vi "HEWH_Agilent_34972A.vi"(8 "error in":errorcluster, 11 "Message Queues out":T2) -> (0 "error out":errorcluster)   [LabVIEW 2023]
uses:
  Tenney/support/Message Queue/All Message Queues.ctl
  Tenney/support/Message Queue/Message Cluster.ctl
  Type Definitions/HEWH Agilent Data.ctl
  Type Definitions/HEWH Full Station IDs.ctl
  FVIR and LDO/support/Message Queue/Enqueue Message (Single).vi
  FVIR and LDO/support/Message Queue/Message Queue.lvlib
  Drivers/Agilent 34972/Agilent 34970.lvlib
  <vilib>/Utility/error.llb/whitespace.ctl
  Tenney/support/Message Queue/Tenney Message Queue.lvlib
panel:
  out "Debug":string[](array[string])
  in  "Debug":bool
  out "Agilent Data":T1
  out "Analog Channel-List":string
  out "Loop Count":i32
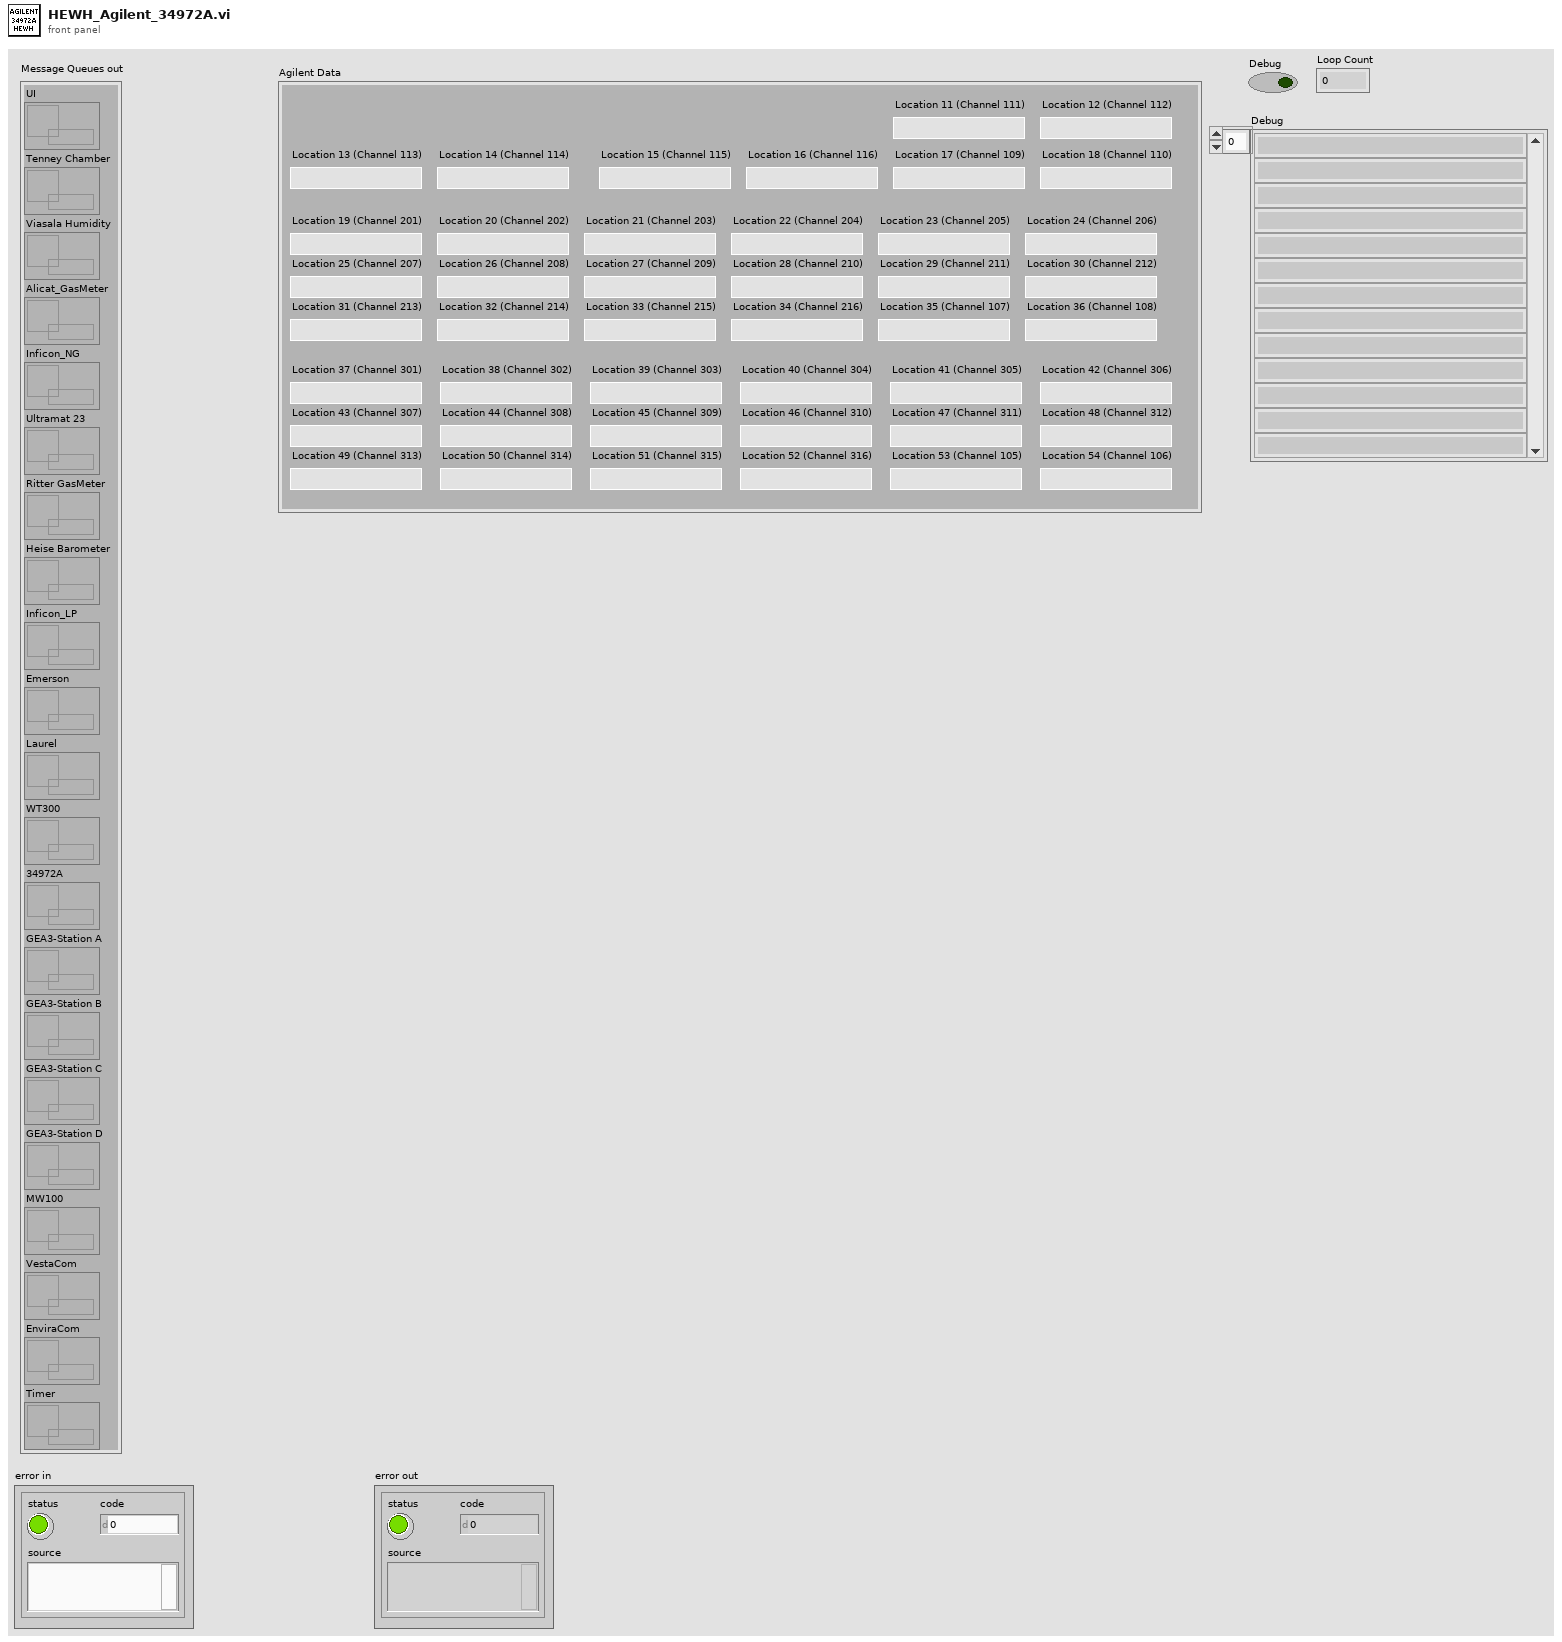
[diagram p1: front panel]
types:
  T1 = typedef "HEWH Agilent Data.ctl" = cluster{"Location 11 (Channel 111)":dbl, "Location 12 (Channel 112)":dbl, "Location 13 (Channel 113)":dbl, "Location 14 (Channel 114)":dbl, "Location 15 (Channel 115)":dbl, "Location 16 (Channel 116)":dbl, "Location 17 (Channel 109)":dbl, "Location 18 (Channel 110)":dbl, "Location 19 (Channel 201)":dbl, "Location 20 (Channel 202)":dbl, "Location 21 (Channel 203)":dbl, "Location 22 (Channel 204)":dbl, "Location 23 (Channel 205)":dbl, "Location 24 (Channel 206)":dbl, "Location 25 (Channel 207)":dbl, "Location 26 (Channel 208)":dbl, "Location 27 (Channel 209)":dbl, "Location 28 (Channel 210)":dbl, "Location 29 (Channel 211)":dbl, "Location 30 (Channel 212)":dbl, "Location 31 (Channel 213)":dbl, "Location 32 (Channel 214)":dbl, "Location 33 (Channel 215)":dbl, "Location 34 (Channel 216)":dbl, "Location 35 (Channel 107)":dbl, "Location 36 (Channel 108)":dbl, "Location 37 (Channel 301)":dbl, "Location 38 (Channel 302)":dbl, "Location 39 (Channel 303)":dbl, "Location 40 (Channel 304)":dbl, "Location 41 (Channel 305)":dbl, "Location 42 (Channel 306)":dbl, "Location 43 (Channel 307)":dbl, "Location 44 (Channel 308)":dbl, "Location 45 (Channel 309)":dbl, "Location 46 (Channel 310)":dbl, "Location 47 (Channel 311)":dbl, "Location 48 (Channel 312)":dbl, "Location 49 (Channel 313)":dbl, "Location 50 (Channel 314)":dbl, "Location 51 (Channel 315)":dbl, "Location 52 (Channel 316)":dbl, "Location 53 (Channel 105)":dbl, "Location 54 (Channel 106)":dbl}
  T2 = typedef "Tenney Message Queue.lvlib/All Message Queues.ctl" = cluster{"UI":refnum<queue>, "Tenney Chamber":refnum<queue>, "Viasala Humidity":refnum<queue>, "Alicat_GasMeter":refnum<queue>, "Inficon_NG":refnum<queue>, "Ultramat 23":refnum<queue>, "Ritter GasMeter":refnum<queue>, "Heise Barometer":refnum<queue>, "Inficon_LP":refnum<queue>, "Emerson":refnum<queue>, "Laurel":refnum<queue>, "WT300":refnum<queue>, "34972A":refnum<queue>, "GEA3-Station A":refnum<queue>, "GEA3-Station B":refnum<queue>, "GEA3-Station C":refnum<queue>, "GEA3-Station D":refnum<queue>, "MW100":refnum<queue>, "VestaCom":refnum<queue>, "EnviraCom":refnum<queue>, "Timer":refnum<queue>}
  T3 = typedef "HEWH Full Station IDs.ctl" = enum16{"Default", "1ED", "2ED", "3ED", "4ED", "6A", "6B", "6C", "6D"}
  T4 = typedef "whitespace.ctl" = u16
  T5 = typedef "HEWH RLT Stations.ctl" = cluster{"MW100 Labels_Channels":T6[], "Agilent Labels_Channels":T6[]}
  T6 = typedef "HEWH Label Channel.ctl" = cluster{"Label":string, "Channel":string}
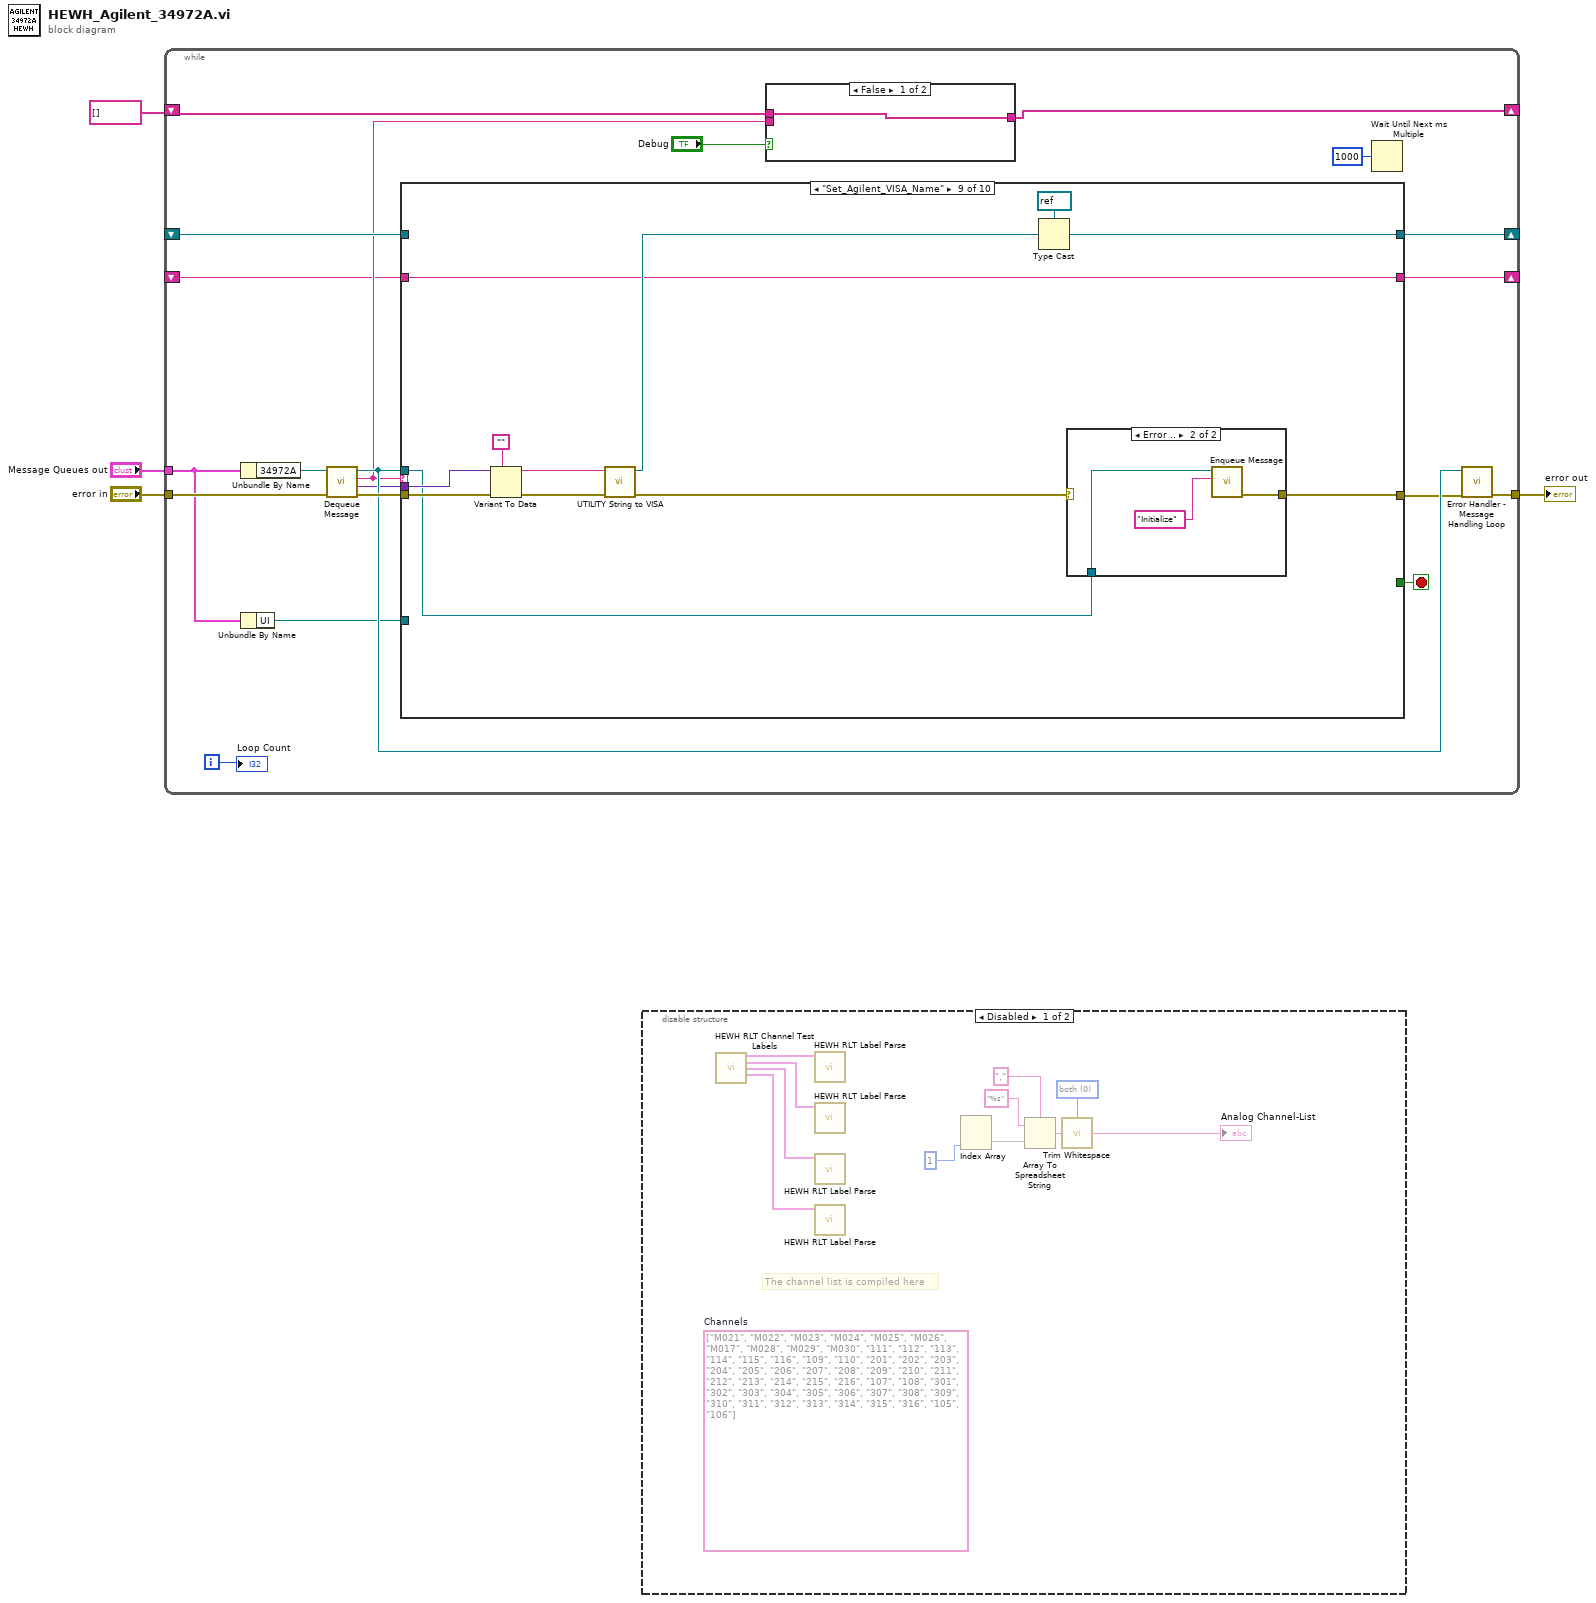
[diagram p0: block diagram]
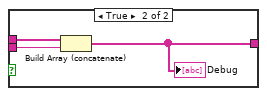
[diagram p3: hidden frame]
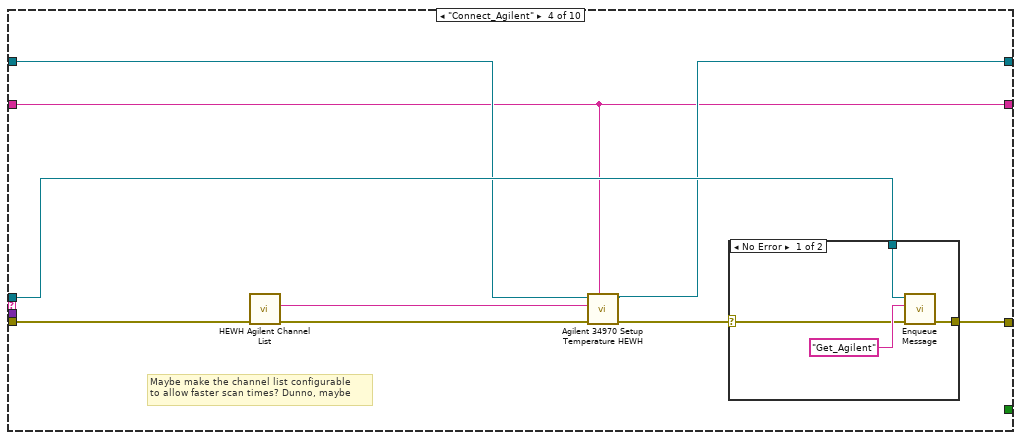
[diagram p7: hidden frame]
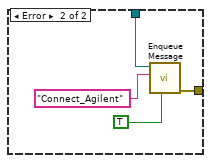
[diagram p8: hidden frame]
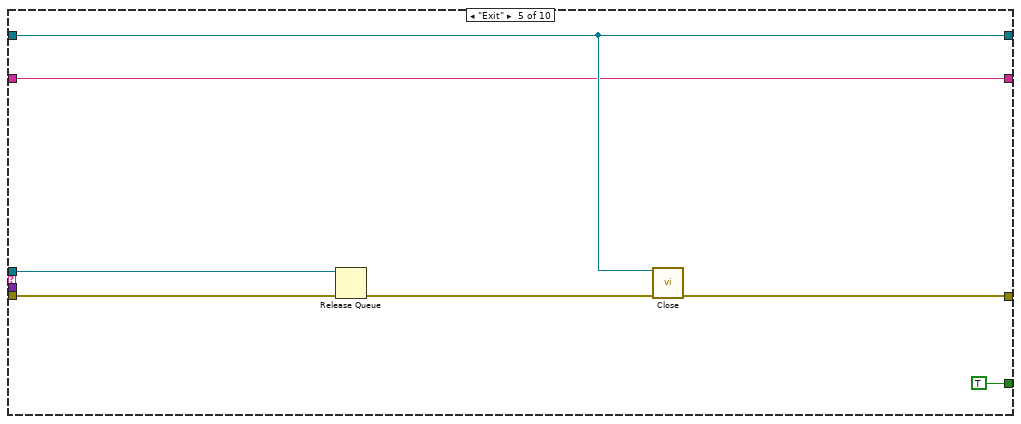
[diagram p9: hidden frame]
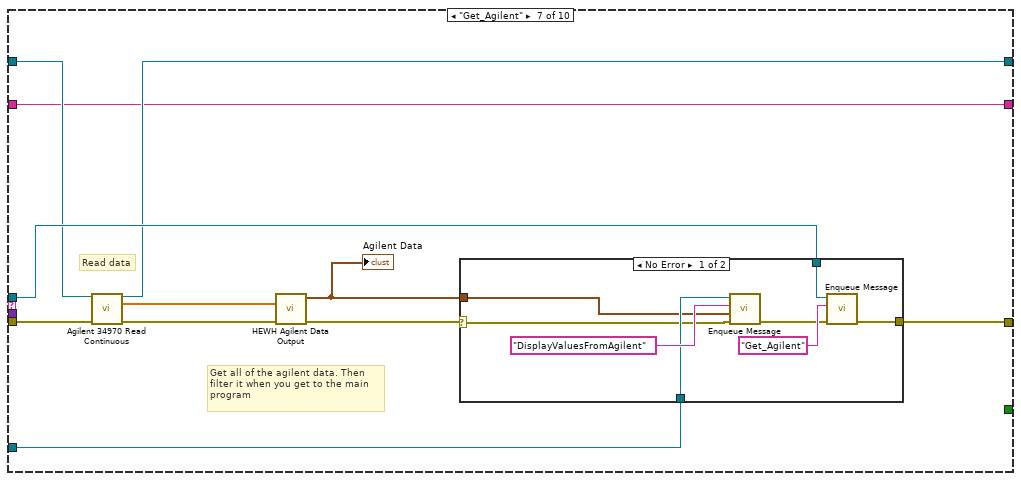
[diagram p11: hidden frame]
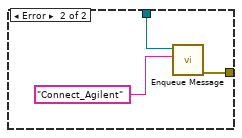
[diagram p12: hidden frame]
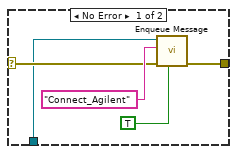
[diagram p14: hidden frame]
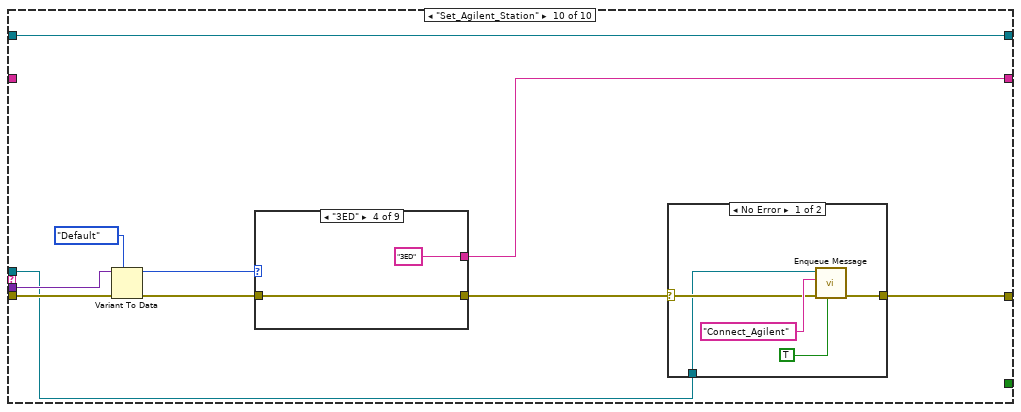
[diagram p15: hidden frame]
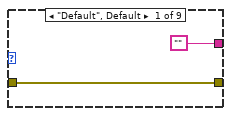
[diagram p16: hidden frame]
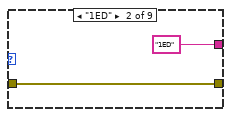
[diagram p17: hidden frame]
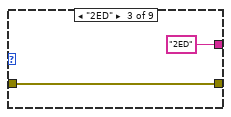
[diagram p18: hidden frame]
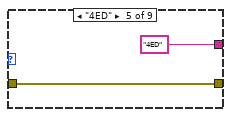
[diagram p19: hidden frame]
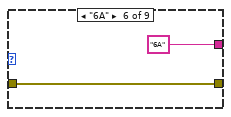
[diagram p20: hidden frame]
diagram:
  n1 = while {
    tunnel: "Message Queues out" -> [w16]
    tunnel: "error in" -> [w23]
    tunnel: [w19] -> w4
    shift-right: [w14] -> _
    shift-left: _ -> [w13]
    shift-right: [w8] -> _
    shift-left: string[] [] -> [w10]
    shift-right: [w6] -> _
    shift-left: _ -> [w5]
    i -> [w12]
    stop <- w21 stop-if-true
    n2 = Unbundle By Name(w16) -> ("34972A"=w24:refnum<queue>)
    n3 = Unbundle By Name(w16) -> ("UI"=w15:refnum<queue>)
    n4 = call "Dequeue Message.vi"("error in (no error)"=w23, "Message Queue"=w24) -> ("error out"=w22:errorcluster, "Message Data"=w7:variant, "Message"=w9:string, "dup Message Queue"=w20:refnum<queue>)  [unwired: 6 in]
    n5 = case shown="\"Set_Agilent_VISA_Name\"" w9 {
      tunnel: w22 -> [w30 w33 w36 w40 w56 w63 w70 w88 w98 w118]
      tunnel: [w30 w33 w36 w46 w58 w63 w74 w88 w92 w116] -> w18
      tunnel: [_ _ _ _ TRUE _ _ _ _ _] -> w21
      tunnel: w20 -> [_ _ _ w45 w60 _ w73 _ w91 w115]
      tunnel: w15 -> [_ _ _ _ _ _ w75 _ _ _]
      tunnel: [w31 w34 w37 w44 w57 w64 w71 w89 w93 w119] -> w14
      tunnel: w13 -> [w31 w34 w37 w39 w57 w64 w72 w89 _ w119]
      tunnel: w7 -> [_ _ _ _ _ _ _ _ w97 w117]
      tunnel: [w29 w32 w35 w38 w55 w62 w65 w87 w90 w110] -> w6
      tunnel: w5 -> [w29 w32 w35 w38 w55 w62 w65 w87 w90 _]
      frame "---------- Setup ----------" {
      }
      frame Default {
      }
      frame "Initialize" {
      }
      frame "Connect_Agilent" {
        # "Maybe make the channel list configurable\nto allow faster scan times? Dunno, maybe"
        n6 = call "HEWH Agilent Channel List.vi"("error in (no error)"=w40) -> ("error out"=w43:errorcluster, "Analog Channel-List"=w42:string)  [unwired: 9 in]
        n7 = call "Agilent 34970 Setup Temperature HEWH.vi"("Station"=w38, "Error In"=w43, "Agilent Channel Input"=w42, "VISA Refnum in"=w39) -> ("Error Out"=w41:errorcluster, "VISA Resource Name Out"=w44:refnum<visa-resource-name>)  [unwired: 6 in]
        n8 = case shown="No Error" w41 {
          selector: w41 -> [w47 _]
          tunnel: [w49 w52] -> w46
          tunnel: w45 -> [w48 w51]
          frame No Error {
            n9 = call-poly "Enqueue Message.vi"("error in (no error)"=w47, "Message"="Get_Agilent", "Message Queue"=w48) -> ("error out"=w49:errorcluster)  [unwired: 7 in, 1 out]
          }
          frame Error {
            n10 = call-poly "Enqueue Message.vi"("Priority Message? (F)"=TRUE, "Message"="Connect_Agilent", "Message Queue"=w51) -> ("error out"=w52:errorcluster)  [unwired: 7 in, 1 out]
          }
        }
      }
      frame "Exit" {
        n11 = Release Queue(queue=w60, error in (no error)=w56) -> (error out=w59:errorcluster)  [unwired: 1 in, 2 out]
        n12 = call "Close.vi"("VISA Resource Name"=w57, "error in (no error)"=w59) -> ("error out"=w58:errorcluster)  [unwired: 13 in]
      }
      frame "---------- Data Collection ----------" {
      }
      frame "Get_Agilent" {
        # "Get all of the agilent data. Then\nfilter it when you get to the main\nprogram"
        # "Read data"
        n13 = call "Agilent 34970 Read Continuous.vi"("VISA Resource Name"=w72, "error in (no error)"=w70) -> ("VISA resource name out"=w71:refnum<visa-resource-name>, "Output Array"=w67:dbl[], "error out"=w68:errorcluster)  [unwired: 10 in, 1 out]
        n14 = call "HEWH Agilent Data Output.vi"("error in (no error)"=w68, "Output Array in"=w67) -> ("error out"=w66:errorcluster, "Agilent Data"=w69:T1)  [unwired: 8 in]
        "Agilent Data" <- w69
        n15 = case shown="No Error" w66 {
          selector: w66 -> [w76 _]
          tunnel: w75 -> [w82 _]
          tunnel: [w79 w85] -> w74
          tunnel: w73 -> [w78 w84]
          tunnel: w69 -> [w77 _]
          frame No Error {
            n16 = call-poly "Enqueue Message.vi"("error in (no error)"=w76, "Message Data"=w77, "Message"="DisplayValuesFromAgilent", "Message Queue"=w82) -> ("error out"=w80:errorcluster)  [unwired: 6 in, 1 out]
            n17 = call-poly "Enqueue Message.vi"("error in (no error)"=w80, "Message"="Get_Agilent", "Message Queue"=w78) -> ("error out"=w79:errorcluster)  [unwired: 7 in, 1 out]
          }
          frame Error {
            n18 = call-poly "Enqueue Message.vi"("Message"="Connect_Agilent", "Message Queue"=w84) -> ("error out"=w85:errorcluster)  [unwired: 8 in, 1 out]
          }
        }
      }
      frame "---------- Events ----------" {
      }
      frame "Set_Agilent_VISA_Name" {
        n19 = Variant To Data(error in=w98, type="", Variant=w97) -> (data=w101:string, error out=w100:errorcluster)
        n20 = call "UTILITY String to VISA.vi"("error in (no error)"=w100, "VISA Name"=w101) -> ("error out"=w95:errorcluster, "VISA resource name out"=w96:refnum<visa-resource-name>)  [unwired: 8 in]
        n21 = Type Cast(type=refnum<visa-resource-name> refnum ("VISA resource name out"), x=w96) -> (*(type *) &x=w93:refnum<visa-resource-name>)
        n22 = case shown="Error .." w95 {
          selector: w95 -> [w104 _]
          tunnel: [w103 w108] -> w92
          tunnel: w91 -> [w102 w107]
          frame No Error {
            n23 = call-poly "Enqueue Message.vi"("Priority Message? (F)"=TRUE, "error in (no error)"=w104, "Message"="Connect_Agilent", "Message Queue"=w102) -> ("error out"=w103:errorcluster)  [unwired: 6 in, 1 out]
          }
          frame Error {
            n24 = call-poly "Enqueue Message.vi"("Message"="Initialize", "Message Queue"=w107) -> ("error out"=w108:errorcluster)  [unwired: 8 in, 1 out]
          }
        }
      }
      frame "Set_Agilent_Station" {
        n25 = Variant To Data(error in=w118, type=HEWH_Full_Station_IDs."Default" ("Full Station ID"), Variant=w117) -> (data=w113:T3, error out=w112:errorcluster)
        n26 = case shown="\"3ED\"" w113 {
          tunnel: w112 -> [w120 w123 w124 w126 w128 w130 w132 w134 w136]
          tunnel: [w120 w123 w124 w126 w128 w130 w132 w134 w136] -> w111
          tunnel: ["" "1ED" "2ED" "3ED" "4ED" "6A" "6B" "6C" "6D"] -> w110
          frame "Default", Default {
          }
          frame "1ED" {
          }
          frame "2ED" {
          }
          frame "3ED" {
          }
          frame "4ED" {
          }
          frame "6A" {
          }
          frame "6B" {
          }
          frame "6C" {
          }
          frame "6D" {
          }
        }
        n27 = case shown="No Error" w111 {
          selector: w111 -> [w140 _]
          tunnel: [w139 errorcluster {"status"=FALSE, "code"=0, "source"=""} ("error out")] -> w116
          tunnel: w115 -> [w138 _]
          frame No Error {
            n28 = call-poly "Enqueue Message.vi"("Priority Message? (F)"=TRUE, "error in (no error)"=w140, "Message"="Connect_Agilent", "Message Queue"=w138) -> ("error out"=w139:errorcluster)  [unwired: 6 in, 1 out]
          }
          frame Error {
          }
        }
      }
    }
    n29 = case shown="False" "Debug" {
      tunnel: w9 -> [_ w28]
      tunnel: w10 -> [w25 w27]
      tunnel: [w25 w26] -> w8
      frame False {
      }
      frame True {
        n30 = Build Array (concatenate)(w27, w28) -> (w26:string[])
        "Debug" <- w26
      }
    }
    n31 = Wait Until Next ms Multiple(millisecond multiple=u32 1000) -> ()  [unwired: 1 out]
    n32 = call "Error Handler - Message Handling Loop.vi"("error in (no error)"=w18, "Message Queue"=w20) -> ("dup error in"=w19:errorcluster)  [unwired: 8 in, 1 out]
    "Loop Count" <- w12
  }
  "error out" <- w4
  n33 = disable-structure shown="Disabled" {
    frame Disabled {
      (unwired) string[][] [["M021", "M022", "M023", "M024", "M025", "M026"], ["M017", "M028", "M029", "M030", "111", "112"], ["113", "114", "115", "116", "109", "110"], ["201", "202", "203", "204", "205", "206"], ["207", "208", "209", "210", "211", "212"], ["213", "214", "215", "216", "107", "108"], ["301", "302", "303", "304", "305", "306"], ["307", "308", "309", "310", "311", "312"], ["313", "314", "315", "316", "105", "106"]]  # Channels
      w149 = T4 0 items=["both", "start of string", "end of string"] ("location (both)")
      # "The channel list is compiled here"
      n34 = call "HEWH RLT Channel Test Labels.vi"() -> ("Station A"=w151:T5, "Station B"=w152:T5, "Station C"=w153:T5, "Station D"=w154:T5)  [unwired: 11 in, 1 out]
      n35 = call "HEWH RLT Label Parse.vi"("Station A"=w151) -> ()  [unwired: 6 in, 5 out]
      n36 = call "HEWH RLT Label Parse.vi"("Station A"=w152) -> ()  [unwired: 6 in, 5 out]
      n37 = call "HEWH RLT Label Parse.vi"("Station A"=w153) -> ()  [unwired: 6 in, 5 out]
      n38 = call "HEWH RLT Label Parse.vi"("Station A"=w154) -> ()  [unwired: 6 in, 5 out]
      n39 = Index Array(index (col)=1 ("disabled index (col)")) -> (element=w148)  [unwired: 2 in]
      n40 = Array To Spreadsheet String(delimiter (Tab)="," ("format string"), array=w148, 3:"%s" ("format string")) -> (spreadsheet string=w146:string)
      n41 = call <vilib>:"Trim Whitespace.vi"("string"=w146, "location (both)"=w149) -> ("trimmed string"=→"Analog Channel-List":string)
    }
    frame Enabled {
    }
  }
